vi "TestFit.vi"   [LabVIEW 2018]
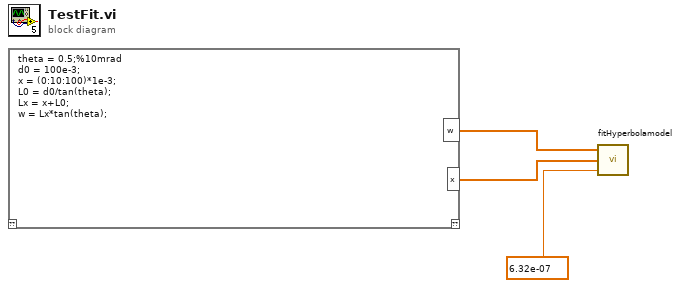
[diagram p0: block diagram]
diagram:
  n1 = script code="theta = 0.5;%10mrad\nd0 = 100e-3;\nx = (0:10:100)*1e-3;\nL0 = d0/tan(theta);\nLx = x+L0;\nw = Lx*tan(theta);"() -> ("w"=w3:dbl[], "x"=w2:dbl[])  [unwired: 1 in, 1 out]
  n2 = call "fitHyperbolamodel.vi"("lambda"=6.32e-07, "Z"=w2, "Wz"=w3) -> ()  [unwired: 2 in, 1 out]
